vi "Create for unparsable.vi"(10 "hostname":string) -> (3 "Generic Network Address out":refnum<class "Generic Network Address.lvclass">)   [LabVIEW 2020, in "NI_WFCN.lvlib" / "Generic Network Address.lvclass"]
doc: "Create a Generic Network Address to represent an invalid or unparsable address."
uses:
  <vilib>/net/WFCN/Addressing/Generic Network Address/Generic Network Address.lvclass
  <vilib>/net/WFCN/Addressing/Generic Network Address/Generic Network Address.lvclass/Generic Network Address.ctl
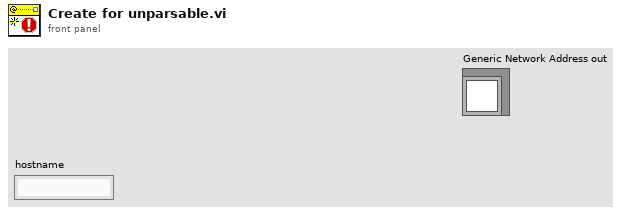
[diagram p1: front panel]
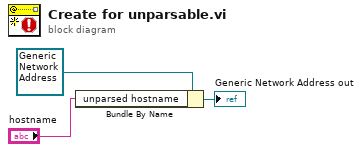
[diagram p0: block diagram]
diagram:
  n1 = Bundle By Name(cluster=refnum<class "Generic Network Address.lvclass"> refnum ("Generic Network Address in"), "unparsed hostname"="hostname") -> (→"Generic Network Address out":refnum<class "Generic Network Address.lvclass">)
